vi "Test-Grabber-Open-Close.vi"() -> ()   [LabVIEW 2014]
uses:
  Robot Actor Framework/Trace/Trace Controller Class/Config.ctl
  Dev Grabber/Dev Grabber Class/Dev Grabber Config.ctl
  <vilib>/Rock Robotics/WPI/Solenoid/WPI_SolenoidChannel.ctl
  Comp Robot/Comp Trace Controller/Comp Trace Controller Class/Comp Trace Controller.lvclass
  Comp Robot/Comp Pressure/Comp Pressure Class/Comp Pressure.lvclass
  Dev Grabber/Dev Grabber Class/Dev Grabber.lvclass
  <vilib>/ActorFramework/Message Enqueuer/Message Enqueuer.lvclass/Message Enqueuer.ctl
  <vilib>/ActorFramework/Message Enqueuer/Enqueue.vi
  <vilib>/ActorFramework/Message Priority Queue/Priority Enqueue.vi
  Robot/Grabber/Grabber Messages/Close Arms Msg/Close Arms Msg.lvclass
  Robot/Grabber/Grabber Messages/Open Arms Msg/Open Arms Msg.lvclass
  <vilib>/ActorFramework/Stop Msg/Stop Msg.lvclass
  <vilib>/ActorFramework/Actor/Actor.lvclass
  Robot Actor Framework/Trace/Trace Controller Class/Trace Controller.lvclass
panel:
  in  "Open":bool=TRUE
  in  "Dev Grabber Config":T1={"PCM CAN ID"=3, "Forward Solenoid Channel"=enum."Solenoid 0", "Reverse Solenoid Channel"=enum."Solenoid 1", "Left Motor CAN ID"=13, "Right Motor CAN ID"=8, "Left Motor Invert"=TRUE, "Right Motor Invert"=FALSE}
  out "Motors error out":errorcluster
  in  "stop":bool
  in  "Config":T3={"Folder Pattern"="/media/sd%s1", "Starting Letter Position"=1, "Min Free Space (MB)"=50.0, "Max Folders to Check"=10, "Trace Level"=enum."Debug"} {"Min Free Space (MB)" format="%#_13g"}
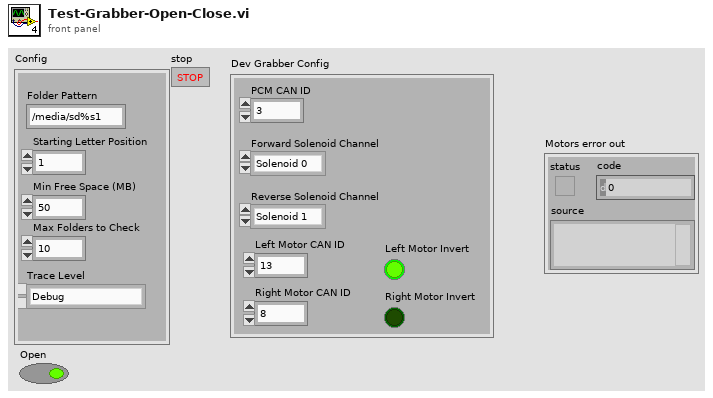
[diagram p1: front panel]
types:
  T1 = typedef "Dev Grabber.lvlib/Dev Grabber.lvclass/Dev Grabber Config.ctl" = cluster{"PCM CAN ID":u8, "Forward Solenoid Channel":T2, "Reverse Solenoid Channel":T2, "Left Motor CAN ID":u8, "Right Motor CAN ID":u8, "Left Motor Invert":bool, "Right Motor Invert":bool}
  T2 = typedef "WPI_SolenoidChannel.ctl" = enum8{"Solenoid 0", "Solenoid 1", "Solenoid 2", "Solenoid 3", "Solenoid 4", "Solenoid 5", "Solenoid 6", "Solenoid 7", "Invalid"}
  T3 = typedef "Robot Actor Framework.lvlib/Trace.lvlib/Trace Controller.lvclass/Config.ctl" = cluster{"Folder Pattern":string, "Starting Letter Position":i32, "Min Free Space (MB)":dbl, "Max Folders to Check":u32, "Trace Level":enum16{"Critical", "Error", "Warning", "Informational", "Debug"}}
  T4 = enum16{"Critical", "Error", "Warning", "Informational", "Debug"}
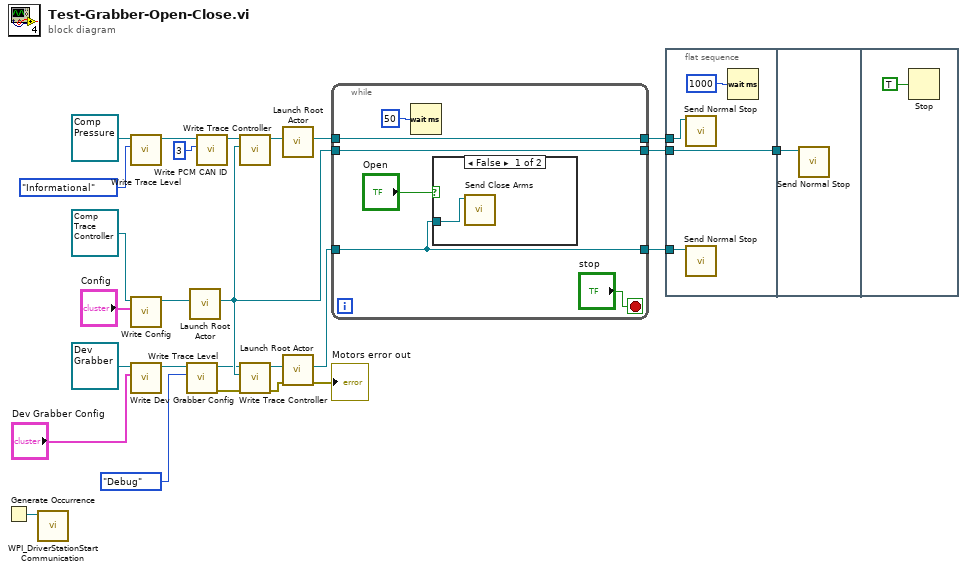
[diagram p0: block diagram]
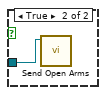
[diagram p2: hidden frame]
diagram:
  n1 = Generate Occurrence() -> (w22:refnum<k4>)
  n2 = call <vilib>:"WPI_DriverStationStart Communication.vi"("occurrence"=w22) -> ()  [unwired: 1 in, 10 out]
  n3 = call-dynamic "Write Trace Level.vi"("Trace Level"=T4."Informational", "System Actor in"=refnum<class "Comp Pressure.lvclass"> refnum ("Comp Pressure.lvlib:Comp Pressure.lvclass")) -> ("System Actor out"=w13:refnum<class "Comp Pressure.lvclass">)  [unwired: 8 in, 1 out]
  n4 = call-dynamic "Write Config.vi"("Config"="Config", "Trace Controller in"=refnum<class "Comp Trace Controller.lvclass"> refnum ("Comp Trace Controller.lvlib:Comp Trace Controller.lvclass")) -> ("Trace Controller out"=w24:refnum<class "Comp Trace Controller.lvclass">)  [unwired: 8 in, 1 out]
  n5 = call-dynamic "Write Dev Grabber Config.vi"("Dev Grabber Config"="Dev Grabber Config", "Dev Grabber in"=refnum<class "Dev Grabber.lvclass"> refnum ("Dev Grabber.lvlib:Dev Grabber.lvclass")) -> ("Dev Grabber out"=w2:refnum<class "Dev Grabber.lvclass">)  [unwired: 8 in, 1 out]
  n6 = call-dynamic "Write Trace Level.vi"("Trace Level"=T4."Debug", "System Actor in"=w2) -> ("error out"=w4:errorcluster, "System Actor out"=w5:refnum<class "Dev Grabber.lvclass">)  [unwired: 8 in]
  n7 = call <vilib>:"Launch Root Actor.vi"("Actor"=w24) -> ("Actor's Enqueuer"=w9:refnum<class "Message Enqueuer.lvclass">)  [unwired: 9 in, 1 out]
  n8 = call-dynamic "Write PCM CAN ID.vi"("PCM CAN ID"=u8 3, "Comp Pressure in"=w13) -> ("Comp Pressure out"=w11:refnum<class "Comp Pressure.lvclass">)  [unwired: 8 in, 1 out]
  n9 = call-dynamic "Write Trace Controller.vi"("Trace Controller"=w9, "System Actor in"=w11) -> ("System Actor out"=w10:refnum<class "Comp Pressure.lvclass">)  [unwired: 8 in, 1 out]
  n10 = call-dynamic "Write Trace Controller.vi"("error in (no error)"=w4, "Trace Controller"=w9, "System Actor in"=w5) -> ("error out"=w16:errorcluster, "System Actor out"=w17:refnum<class "Dev Grabber.lvclass">)  [unwired: 7 in]
  n11 = call <vilib>:"Launch Root Actor.vi"("Actor"=w10) -> ("Actor's Enqueuer"=w8:refnum<class "Message Enqueuer.lvclass">)  [unwired: 9 in, 1 out]
  n12 = call <vilib>:"Launch Root Actor.vi"("error in (no error)"=w16, "Actor"=w17) -> ("error out"=→"Motors error out":errorcluster, "Actor's Enqueuer"=w21:refnum<class "Message Enqueuer.lvclass">)  [unwired: 8 in]
  n13 = while {
    tunnel: w9 -> [w30]
    tunnel: [w30] -> w23
    tunnel: w21 -> [w27]
    tunnel: [w27] -> w19
    tunnel: w8 -> [w29]
    tunnel: [w29] -> w7
    stop <- "stop" stop-if-true
    n14 = Wait (ms)(milliseconds to wait=u32 50) -> ()  [unwired: 1 out]
    n15 = case shown="False" "Open" {
      tunnel: w27 -> [w33 w34]
      frame False {
        n16 = call "Send Close Arms.vi"("Message Enqueuer"=w33) -> ()  [unwired: 9 in, 2 out]
      }
      frame True {
        n17 = call "Send Open Arms.vi"("Message Enqueuer"=w34) -> ()  [unwired: 9 in, 2 out]
      }
    }
  }
  n18 = flat-sequence {
    tunnel: w23 -> [w38]
    tunnel: [w38] -> w20
    tunnel: w19 -> [w37]
    tunnel: w7 -> [w35]
    tunnel: w20 -> [w39]
    frame #0 {
      n19 = call <vilib>:"Send Normal Stop.vi"("Message Enqueuer"=w35) -> ()  [unwired: 10 in, 1 out]
      n20 = call <vilib>:"Send Normal Stop.vi"("Message Enqueuer"=w37) -> ()  [unwired: 10 in, 1 out]
      n21 = Wait (ms)(milliseconds to wait=u32 1000) -> ()  [unwired: 1 out]
    }
    frame #1 {
      n22 = call <vilib>:"Send Normal Stop.vi"("Message Enqueuer"=w39) -> ()  [unwired: 10 in, 1 out]
    }
    frame #2 {
      n23 = Stop(stop? (T)=TRUE) -> ()
    }
  }
